vi "ModifyClassAttribute1.vi"(1 "Lock time (ms)":u32, 2 "timeout in ms (-1)":i32=-1, 3 "Only unlock data? (F)":bool, 4 "Unlock data if error? (T)":bool=TRUE, 5 "error in (no error)":errorcluster, 7 "status":bool) -> (16 "timeout":bool, 17 "created new":bool, 19 "error out":errorcluster)   [LabVIEW 2020, in "G#SubClass2.lvclass"]
uses:
  G#SubClass2.lvclass
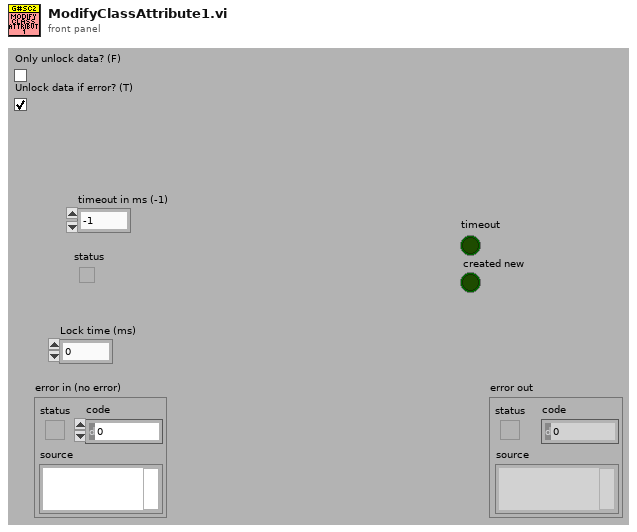
[diagram p1: front panel]
types:
  T1 = typedef "G#SubClass2.lvclass/ClassAttributes.ctl" = cluster{"Base class":T2, "SubClassAttr":i32}
  T2 = typedef "G#BaseClass2.lvclass/ClassAttributes.ctl" = cluster{"ClassAttr":i32}
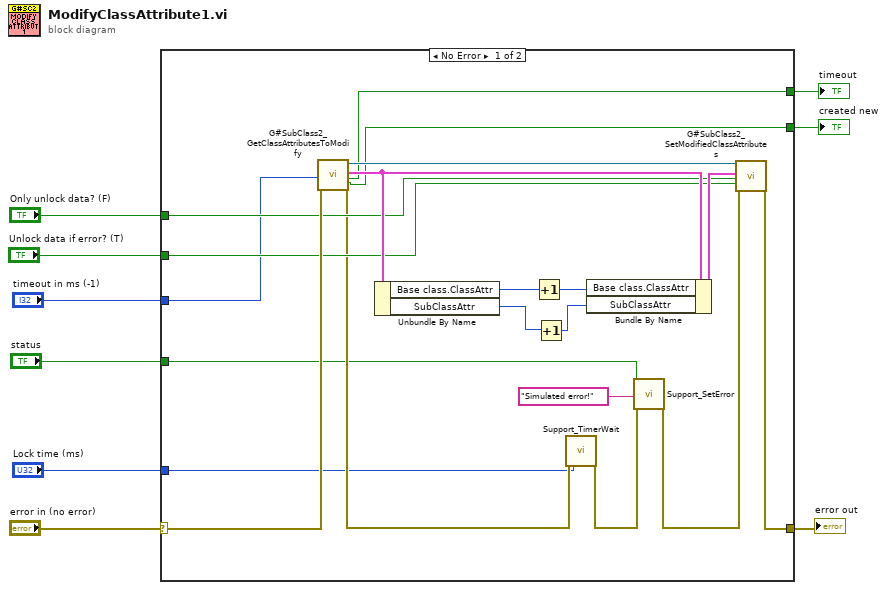
[diagram p0: block diagram]
diagram:
  n1 = case shown="No Error" "error in (no error)" {
    selector: "error in (no error)" -> [w26 w30]
    tunnel: [w27 w30] -> w8
    tunnel: "Only unlock data? (F)" -> [w20 _]
    tunnel: "Unlock data if error? (T)" -> [w19 _]
    tunnel: "Lock time (ms)" -> [w17 _]
    tunnel: "status" -> [w13 _]
    tunnel: "timeout in ms (-1)" -> [w12 _]
    tunnel: [w11 _] -> w2
    tunnel: [w10 _] -> w1
    frame No Error {
      n2 = call "G#SubClass2_GetClassAttributesToModify.vi"("timeout in ms (-1)"=w12, "error in (no error)"=w26) -> ("reference out"=w28:refnum<class "G#SubClass2.lvclass">, "class attributes"=w25:T1, "timeout"=w11:bool, "created new"=w10:bool, "error out"=w18:errorcluster)  [unwired: 12 in, 1 out]
      n3 = Unbundle By Name(w25) -> ("Base class.ClassAttr"=w23:i32, "SubClassAttr"=w22:i32)
      n4 = Increment(x=w23) -> (x+1=w24:i32)
      n5 = Increment(x=w22) -> (x+1=w21:i32)
      n6 = call "Support_TimerWait.vi"("error in (no error)"=w18, "milliseconds to wait"=w17) -> ("error out"=w16:errorcluster)  [unwired: 17 in]
      n7 = Bundle By Name(cluster=w25, "Base class.ClassAttr"=w24, "SubClassAttr"=w21) -> (w29:T1)
      n8 = call "Support_SetError.vi"("status"=w13, "source"="Simulated error!", "error in (no error)"=w16) -> ("error out"=w15:errorcluster)  [unwired: 16 in]
      n9 = call "G#SubClass2_SetModifiedClassAttributes.vi"("reference in"=w28, "attributes"=w29, "Only unlock data? (F)"=w20, "Unlock data if error? (T)"=w19, "error in (no error)"=w15) -> ("error out"=w27:errorcluster)  [unwired: 13 in, 1 out]
    }
    frame Error {
    }
  }
  "error out" <- w8
  "timeout" <- w2
  "created new" <- w1
